vi "Format LogRecord.vi"(8 "error in":errorcluster, 10 "LogRecord":refnum<class "LogRecord.lvclass">, 11 "Formatter in":refnum<class "Formatter.lvclass">) -> (0 "error out":errorcluster, 2 "LogLine":string)   [LabVIEW 2016, in "hse-logger.lvlib" / "Formatter.lvclass"]
doc: "Format the Log Record with a Format String. Each line ends with a newline character."
uses:
  Formatter.lvclass
  LogRecord/LogRecord.lvclass
  Formatter.lvclass/Formatter.ctl
  LogRecord/LogRecord.lvclass/LogRecord.ctl
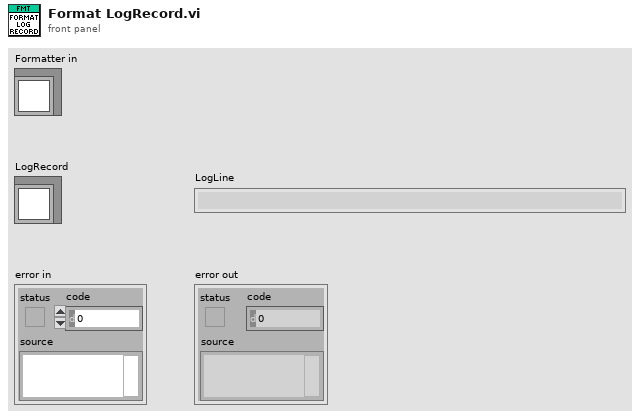
[diagram p1: front panel]
types:
  T1 = typedef "hse-logger.lvlib/LogLevel.ctl" = enum16{"DEBUG", "INFO", "WARNING", "ERROR", "CRITICAL"}
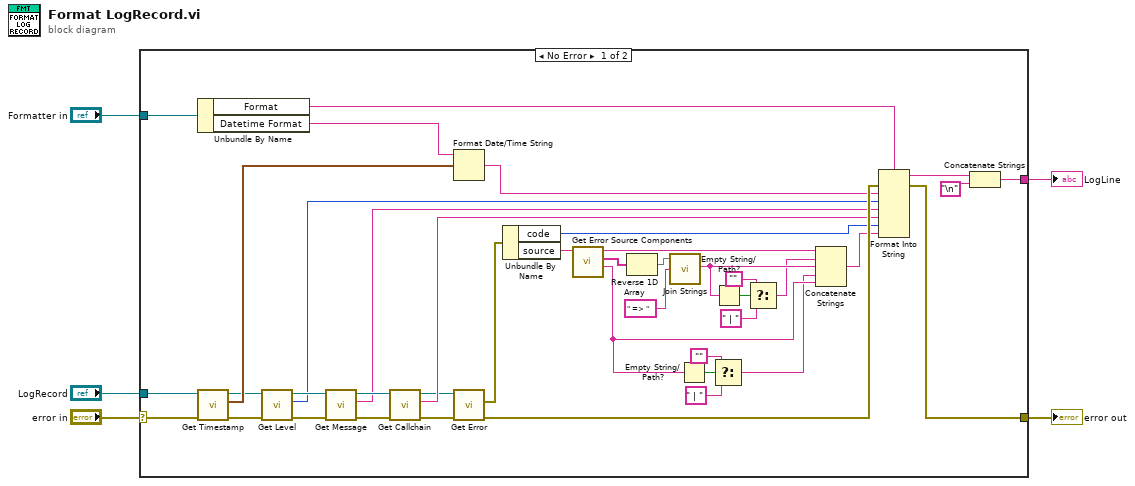
[diagram p0: block diagram]
diagram:
  n1 = case shown="No Error" "error in" {
    selector: "error in" -> [w39 w47]
    tunnel: [w38 w47] -> w4
    tunnel: "Formatter in" -> [w35 _]
    tunnel: "LogRecord" -> [w32 _]
    tunnel: [w28 _] -> w1
    frame No Error {
      n2 = Unbundle By Name(w35) -> ("Format"=w34:string, "Datetime Format"=w30:string)
      n3 = call "Get Timestamp.vi"("error in"=w39, "LogRecord in"=w32) -> ("error out"=w33:errorcluster, "Created"=w31:timestamp, "LogRecord out"=w27:refnum<class "LogRecord.lvclass">)  [unwired: 7 in]
      n4 = call "Get Level.vi"("error in"=w33, "LogRecord in"=w27) -> ("error out"=w44:errorcluster, "Level"=w26:T1, "LogRecord out"=w42:refnum<class "LogRecord.lvclass">)  [unwired: 7 in]
      n5 = call "Get Message.vi"("error in"=w44, "LogRecord in"=w42) -> ("error out"=w45:errorcluster, "Message"=w37:string, "LogRecord out"=w43:refnum<class "LogRecord.lvclass">)  [unwired: 7 in]
      n6 = call "Get Callchain.vi"("error in"=w45, "LogRecord in"=w43) -> ("error out"=w24:errorcluster, "Callchain"=w36:string, "LogRecord out"=w23:refnum<class "LogRecord.lvclass">)  [unwired: 7 in]
      n7 = Format Date/Time String(time format string (%c)=w30, seconds (now)=w31) -> (date/time string=w29:string)  [unwired: 1 in]
      n8 = call "Get Error.vi"("error in"=w24, "LogRecord in"=w23) -> ("error out"=w46:errorcluster, "Error"=w25:errorcluster)  [unwired: 7 in, 1 out]
      n9 = Unbundle By Name(w25) -> ("code"=w41:i32, "source"=w22:string)
      n10 = call "Get Error Source Components.vi"("Error Source String"=w22) -> ("DQMH Error Hint"=w15:string, "Call Chain"=w20:string[], "Error Message"=w21:string)  [unwired: 8 in]
      n11 = Reverse 1D Array(array=w20) -> (reversed array=w16:string[])
      n12 = call <vilib>:"Join Strings.vi"("Separator (,)"=" => " ("string"), "Strings In"=w16) -> ("String"=w7:string)  [unwired: 1 in]
      n13 = Empty String/Path?(string/path=w15) -> (empty?=w14:bool)
      n14 = Select(t="", s=w14, f=" | " ("string")) -> (s? t:f=w11:string)
      n15 = Empty String/Path?(string/path=w7) -> (empty?=w8:bool)
      n16 = Select(t="", s=w8, f=" | " ("string")) -> (s? t:f=w6:string)
      n17 = Concatenate Strings(w21, w6, w7, w11, w15) -> (w19:string)
      n18 = Format Into String(format string=w34, error in=w46, w29, w26, w37, w36, w41, w19) -> (resulting string=w40:string, error out=w38:errorcluster)  [unwired: 1 in]
      n19 = Concatenate Strings(w40, "\n") -> (w28:string)
    }
    frame Error {
    }
  }
  "error out" <- w4
  "LogLine" <- w1
